vi "Write airmass.vi"(8 "error in (no error)":errorcluster, 10 "airmass":dbl=3.0 min=1.0 max=15.0, 11 "AmLimit in":refnum<class "AmLimit.lvclass">) -> (0 "error out":errorcluster, 3 "AmLimit out":refnum<class "AmLimit.lvclass">)   [LabVIEW 2022 SP3, in "TCSDataDefinitions.lvlib" / "TCSCommand.lvlib" / "AmLimit.lvclass"]
uses:
  AmLimit.lvclass
  AmLimit.lvclass/AmLimit.ctl
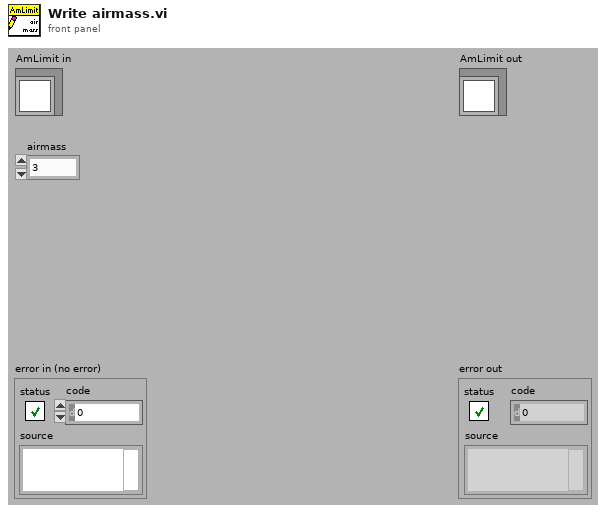
[diagram p1: front panel]
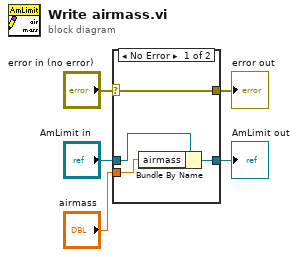
[diagram p0: block diagram]
diagram:
  n1 = case shown="No Error" "error in (no error)" {
    selector: "error in (no error)" -> [w9 w10]
    tunnel: [w9 w10] -> w4
    tunnel: [w7 w11] -> w2
    tunnel: "AmLimit in" -> [w8 w11]
    tunnel: "airmass" -> [w6 _]
    frame No Error {
      n2 = Bundle By Name(cluster=w8, "airmass"=w6) -> (w7:refnum<class "AmLimit.lvclass">)
    }
    frame Error {
    }
  }
  "error out" <- w4
  "AmLimit out" <- w2
